vi "measureCombs_RF.vi"(3 "Read freqs. \nfrom textfile":bool=TRUE, 5 "Cluster":T2={"span"=600000000.0, "rbw"=1000.0, "enableVBW"=FALSE, "vbw"=0.0, "traceLength"=64001, "window"=0, "verticalUnit"=0, "center freq"=300000000.0} {"verticalUnit" items=["SpectrumVerticalUnit_dBm", "SpectrumVerticalUnit_Watt", "SpectrumVerticalUnit_Volt", "SpectrumVerticalUnit_Amp", "SpectrumVerticalUnit_dBmV"]; "window" items=["SpectrumWindow_Kaiser", "SpectrumWindow_Mil6dB", "SpectrumWindow_BlackmanHarris", "SpectrumWindow_Rectangle", "SpectrumWindow_FlatTop", "SpectrumWindow_Hann"]; "traceLength" items=["801"=801, "2401"=2401, "4001"=4001, "8001"=8001, "10401"=10401, "16001"=16001, "32001"=32001, "64001"=64001]}, 7 "RFC/ AFC measurement time":i32=30, 9 "Folder for all data (Don't forget the last slash!)":string) -> (0 "error out":errorcluster={"status"=TRUE, "code"=-1073807346, "source"="VISA Write in Agilent 33XXX Series.lvlib:Error Query.vi->Agilent 33XXX Series.lvlib:Close.vi->closeFncGen_AS.vi->measureCombs_anySet_keepAgilentOpen.vi"})   [LabVIEW 2016]
uses:
  <vilib>/Utility/file.llb/Read Delimited Spreadsheet (DBL).vi
  <vilib>/Utility/file.llb/Write Delimited Spreadsheet (DBL).vi
panel:
  in  "Agilent 33250A address":refnum<visa-resource-name>="GPIB0::4::INSTR"
  in  "Serial Configuration":T1={"Baud Rate"=9600, "Parity"=0, "Data Bits"=8, "Flow Control"=4} {"Flow Control" items=["None", "XON/XOFF", "RTS/CTS", "XON/XOFF & RTS/CTS", "DTR/DSR", "XON/XOFF & DTR/DSR"]; "Data Bits" items=["7"=7, "8"=8]; "Parity" items=["None", "Odd", "Even", "Mark", "Space"]; "Baud Rate" items=["300"=300, "600"=600, "1200"=1200, "2400"=2400, "4800"=4800, "9600"=9600, "19200"=19200]}
  in  "error in":errorcluster
  out "Last saved trace":sgl[](graph)
  in  "stop":bool
  out "RSA error out":errorcluster
  out "Real-time trace":sgl[](graph)
  out "Current set #":i32
  out "Current freq.":dbl=100000.0
  in  "freqs. file":path
  in  "Shuffle?":bool
  in  "Start freq":dbl=1000000.0 format="%0.2e"
  in  "End freq":dbl=2000000.0 format="%0.2e"
  in  "Freq step":i32=100000 format="%.2e"
  out "Duration array":T3(array[cluster])
  in  "Mod shape":enum16{"Triangle", "Sine"}(ring)
  # "consecutive sweeps can be compared\nto check for probe on AFC."
  # "RSA settings"
  # "Suppose you want to collect comb data, first ascending, then descending.\n\nIn Matlab, create a 1xM array \ncontaining all modulation freqs (Hz) in the ascending sequence; then create a 1xN array for the descending case. Note that M != N is fine.\n\nfid= fopen(FILENAME, 'w');\nfprintf(fid,'%d\\t', ARRAY1);\nfprintf(fid,'\\r\\n');\nfprintf(fid,'%d\\t',ARRAY2);\n... \n(for more sets, repeat as needed)\nfclose(fid);\n\nNow find the file you just made:"
  # "Modulation settings"
  # "(zero-indexed)"
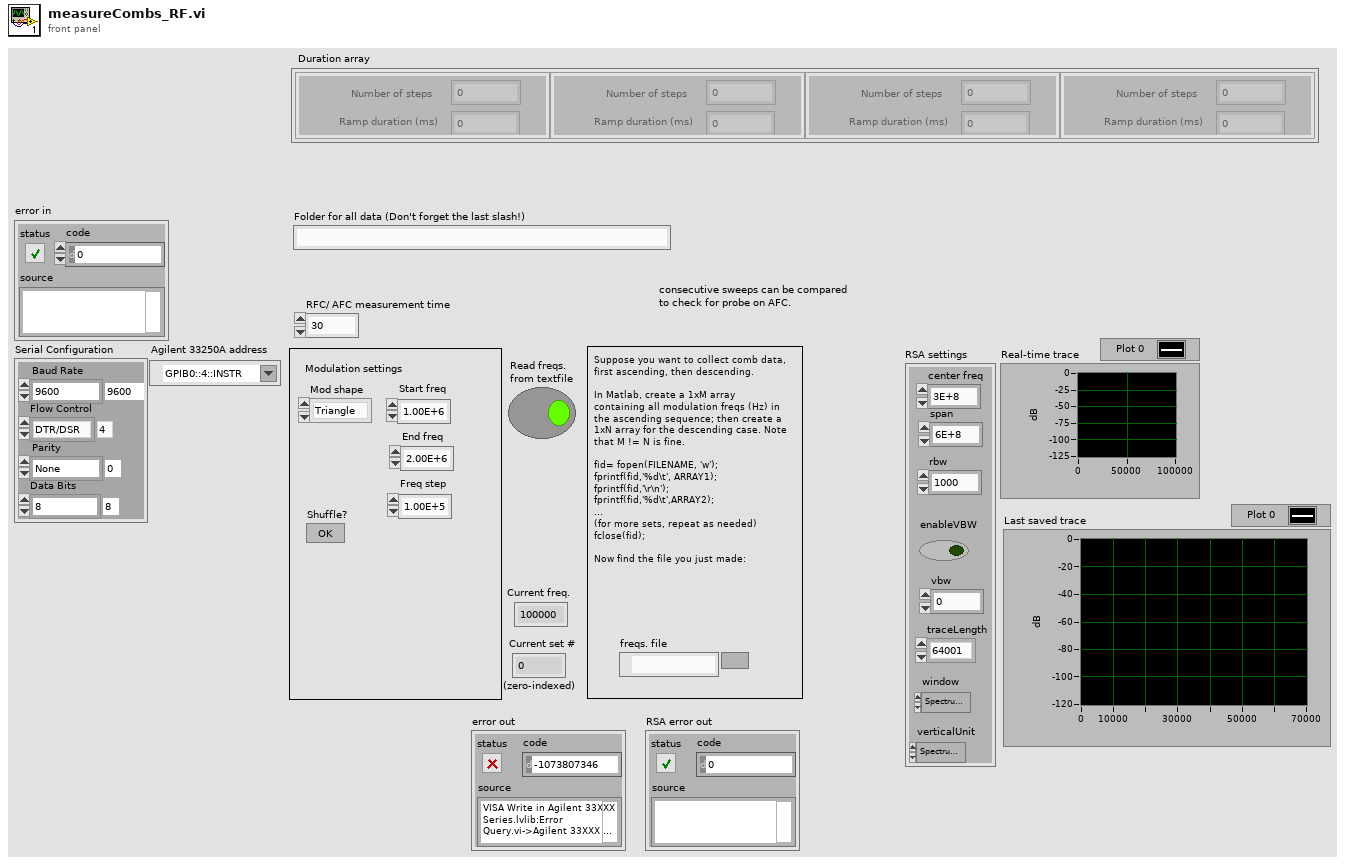
[diagram p1: front panel]
types:
  T1 = cluster{"Baud Rate":u32, "Parity":u16, "Data Bits":u16, "Flow Control":u16}
  T2 = cluster{"span":dbl, "rbw":dbl, "enableVBW":bool, "vbw":dbl, "traceLength":u16, "window":u32, "verticalUnit":u32, "center freq":dbl}
  T3 = cluster{"Number of steps":dbl, "Ramp duration (ms)":dbl}[]
  T4 = cluster{"span":dbl, "rbw":dbl, "enableVBW":bool, "vbw":dbl, "traceLength":u16, "window":u32, "verticalUnit":u32}
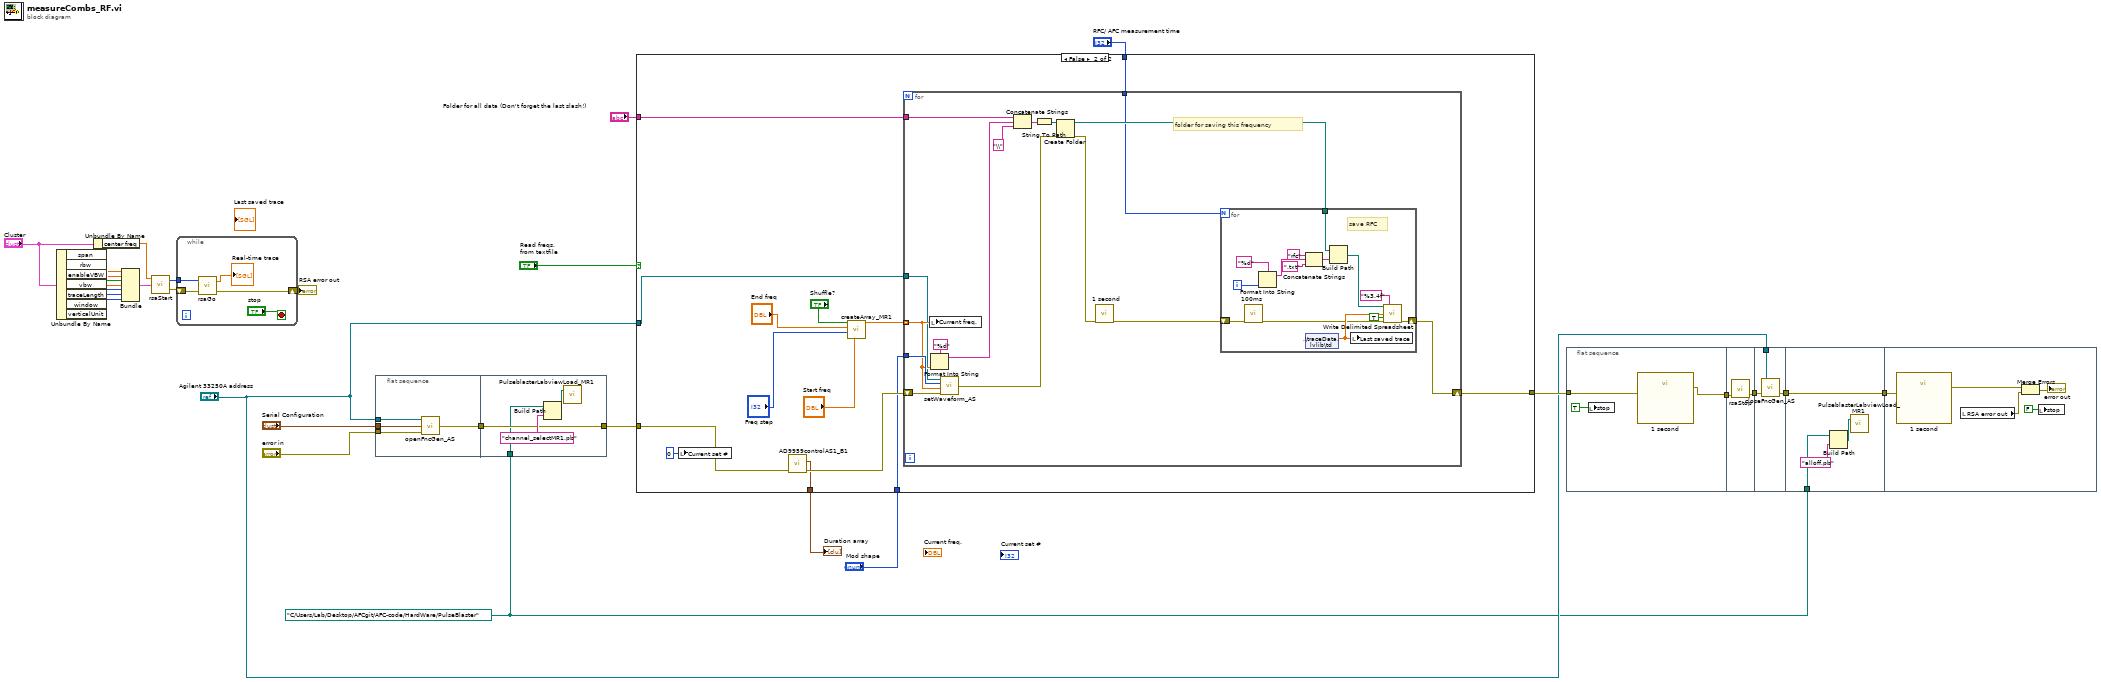
[diagram p0: block diagram]
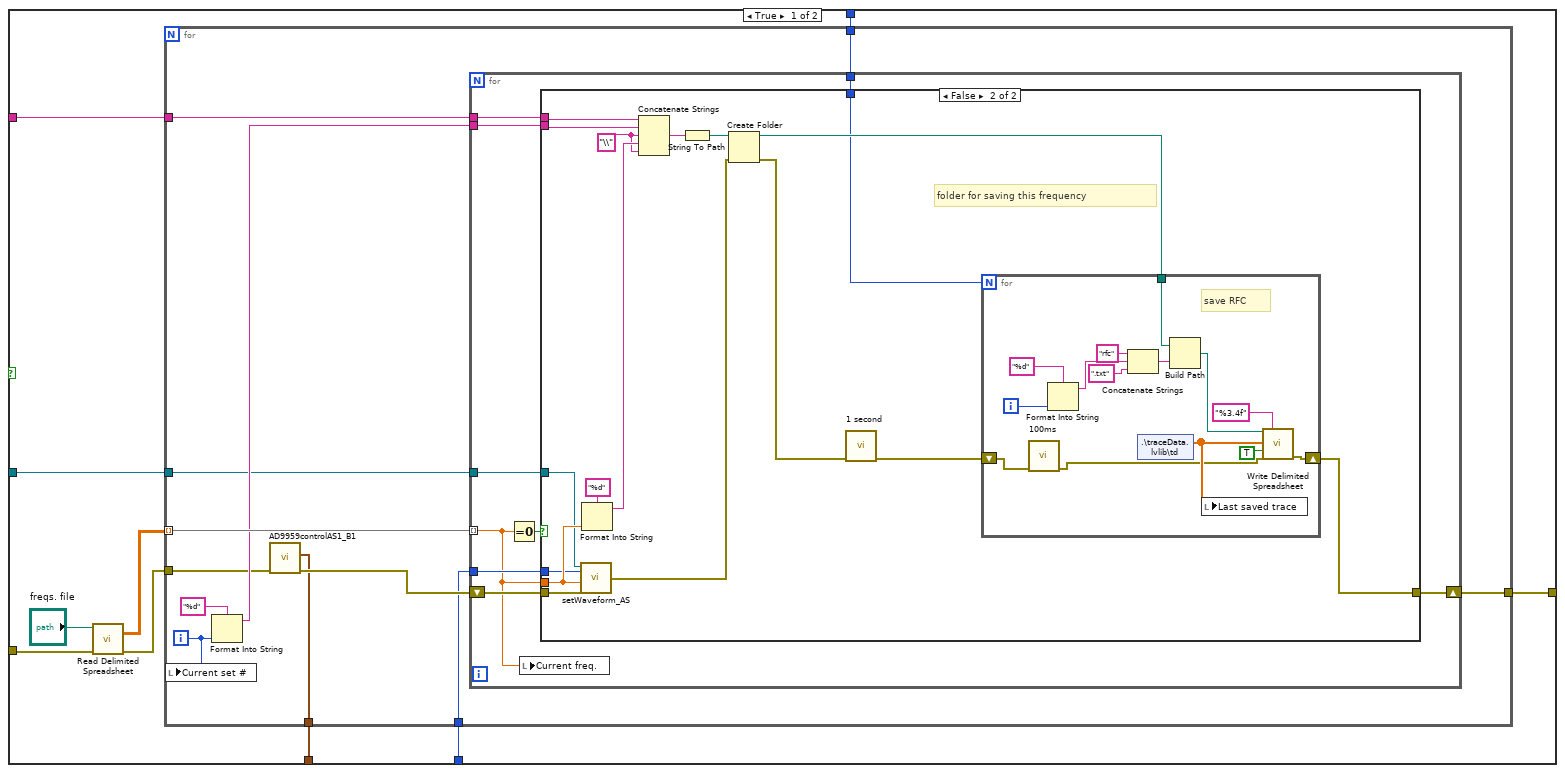
[diagram p2: hidden frame]
diagram:
  w1 = path "C:/Users/Lab/Desktop/AFCgit/AFC-code/HardWare/PulseBlaster" ("base path")
  n1 = Unbundle By Name("Cluster") -> ("span"=w22:dbl, "rbw"=w23:dbl, "enableVBW"=w24:bool, "vbw"=w25:dbl, "traceLength"=w26:u16, "window"=w27:u32, "verticalUnit"=w28:u32)
  n2 = Unbundle By Name("Cluster") -> ("center freq"=w16:dbl)
  n3 = Bundle("span"=w22, "rbw"=w23, "enableVBW"=w24, "vbw"=w25, "traceLength"=w26, "window"=w27, "verticalUnit"=w28) -> (w15:T4)  [unwired: 1 in]
  n4 = call "rsaStart.vi"("Cluster"=w15, "center freq"=w16) -> ("error out"=w13:errorcluster, "traceLength"=w14:u16)  [unwired: 1 in]
  n5 = while {
    tunnel: w14 -> [w34]
    shift-right: [w32] -> w12
    shift-left: w13 -> [w31]
    stop <- "stop" stop-if-true
    n6 = call "rsaGo.vi"("error in"=w31, "Trace length"=w34) -> ("error out"=w32:errorcluster, "traceData out"=→"Real-time trace":sgl[])  [unwired: 1 in]
  }
  "RSA error out" <- w12
  n7 = flat-sequence {
    tunnel: "error in" -> [w38]
    tunnel: "Serial Configuration" -> [w37]
    tunnel: "Agilent 33250A address" -> [w36]
    tunnel: [w35] -> w3
    tunnel: [w40] -> w2
    tunnel: w3 -> [w40]
    tunnel: w1 -> [w39]
    frame #0 {
      n8 = call "openFncGen_AS.vi"("error in (no error)"=w38, "Serial Configuration"=w37, "VISA resource name"=w36) -> ("error out"=w35:errorcluster)
    }
    frame #1 {
      n9 = Build Path(base path=w39, name or relative path="channel_selectMR1.pb") -> (appended path=w42:path)
      n10 = call "PulseblasterLabviewLoad_MR1.vi"("Input file"=w42) -> ()  [unwired: 1 in, 2 out]
    }
  }
  n11 = case shown="False" "Read freqs. \nfrom textfile" {
    tunnel: "Folder for all data (Don't forget the last slash!)" -> [w52 w119]
    tunnel: "RFC/ AFC measurement time" -> [w51 w117]
    tunnel: w2 -> [w49 w111]
    tunnel: "Mod shape" -> [w46 w110]
    tunnel: [w45 w109] -> w17
    tunnel: [w44 w107] -> w29
    tunnel: "Agilent 33250A address" -> [w43 w106]
    frame True {
      n12 = call-poly <vilib>:"Read Delimited Spreadsheet.vi"("file path (dialog if empty)"="freqs. file", "error in (no error)"=w49) -> ("all rows"=w48:dbl[][], "error out"=w47:errorcluster)  [unwired: 8 in, 4 out]
      n13 = for {
        tunnel: [w64] -> w44
        tunnel: w52 -> [w63]
        tunnel: w51 -> [w61]
        tunnel: w48 -> [w60] mode=indexing
        tunnel: w47 -> [w57]
        tunnel: w46 -> [w56]
        tunnel: [w55] -> w45
        tunnel: w43 -> [w53]
        i -> [w54]
        n14 = local write "Current set #"(w54) -> ()
        n15 = Format Into String(format string="%d", w54) -> (resulting string=w58:string)  [unwired: 2 in, 1 out]
        n16 = call "AD9959controlAS1_B1.vi"("error in (no error)"=w57) -> ("error out"=w62:errorcluster, "Duration array"=w55:T3)  [unwired: 9 in]
        n17 = for {
          tunnel: w60 -> [w66] mode=indexing
          tunnel: w56 -> [w73]
          shift-right: [w72] -> w64
          shift-left: w62 -> [w71]
          tunnel: w63 -> [w68]
          tunnel: w61 -> [w70]
          tunnel: w58 -> [w69]
          tunnel: w53 -> [w65]
          n18 = Equal To 0?(x=w66) -> (x = 0?=w67:bool)
          n19 = local write "Current freq."(w66) -> ()
          n20 = case shown="False" w67 {
            tunnel: w73 -> [_ w79]
            tunnel: [w74 w75] -> w72
            tunnel: w71 -> [w74 w81]
            tunnel: w70 -> [_ w89]
            tunnel: w69 -> [_ w84]
            tunnel: w68 -> [_ w85]
            tunnel: w66 -> [_ w80]
            tunnel: w65 -> [_ w78]
            frame True {
            }
            frame False {
              w87 = "\\" ("string")
              # "folder for saving this frequency"
              n21 = call "setWaveform_AS.vi"("error in (no error)"=w81, "Frequency (1000 Hz)"=w80, "Enum"=w79, "VISA resource name"=w78) -> ("error out"=w76:errorcluster)
              n22 = Format Into String(format string="%d", w80) -> (resulting string=w88:string)  [unwired: 2 in, 1 out]
              n23 = Concatenate Strings(w85, w84, w87, w88, w87) -> (w83:string)
              n24 = String To Path(string=w83) -> (path=w90:path)
              n25 = Create Folder(path (use dialog)=w90, error in=w76) -> (created path=w91:path, error out=w77:errorcluster)  [unwired: 1 in, 1 out]
              n26 = call "1 second"("error in (no error)"=w77) -> ("error out"=w82:errorcluster)  [unwired: 10 in]
              n27 = for {
                N: w89 -> [_]
                shift-right: [w104] -> w75
                shift-left: w82 -> [w93]
                tunnel: w91 -> [w96]
                i -> [w100]
                # "save RFC"
                n28 = call "100ms"("error in (no error)"=w93) -> ("error out"=w92:errorcluster)  [unwired: 10 in]
                n29 = Format Into String(format string="%d", w100) -> (resulting string=w99:string)  [unwired: 2 in, 1 out]
                n30 = Concatenate Strings("rfc" ("string"), w99, ".txt" ("string")) -> (w98:string)
                n31 = shared-variable ".\\traceData.lvlib\\td"() -> (w94:dbl[])  [unwired: 1 in, 1 out]
                n32 = Build Path(base path=w96, name or relative path=w98) -> (appended path=w103:path)
                n33 = local write "Last saved trace"(w94) -> ()
                n34 = call-poly <vilib>:"Write Delimited Spreadsheet.vi"("file path (dialog if empty)"=w103, "format (%.3f)"="%3.4f", "1D data"=w94, "append to file? (new file:F)"=TRUE, "error in (no error)"=w92) -> ("error out"=w104:errorcluster)  [unwired: 9 in, 1 out]
              }
            }
          }
        }
      }
    }
    frame False {
      n35 = local write "Current set #"(0 ("Current set #")) -> ()
      n36 = call "AD9959controlAS1_B1.vi"("error in (no error)"=w111) -> ("error out"=w118:errorcluster, "Duration array"=w109:T3)  [unwired: 9 in]
      n37 = call "createArray_MR1.vi"("Start freq"="Start freq", "Freq step"="Freq step", "End freq"="End freq", "Shuffle?"="Shuffle?") -> ("Riffled {X}"=w112:dbl[])  [unwired: 7 in]
      n38 = for {
        tunnel: w112 -> [w125] mode=indexing
        tunnel: w110 -> [w126]
        shift-right: [w120] -> w107
        shift-left: w118 -> [w127]
        tunnel: w119 -> [w130]
        tunnel: w117 -> [w129]
        tunnel: w106 -> [w124]
        # "folder for saving this frequency"
        n39 = local write "Current freq."(w125) -> ()
        n40 = Format Into String(format string="%d", w125) -> (resulting string=w134:string)  [unwired: 2 in, 1 out]
        n41 = call "setWaveform_AS.vi"("error in (no error)"=w127, "Frequency (1000 Hz)"=w125, "Enum"=w126, "VISA resource name"=w124) -> ("error out"=w121:errorcluster)
        n42 = Concatenate Strings(w130, w134, "\\" ("string")) -> (w132:string)
        n43 = String To Path(string=w132) -> (path=w131:path)
        n44 = Create Folder(path (use dialog)=w131, error in=w121) -> (created path=w133:path, error out=w123:errorcluster)  [unwired: 1 in, 1 out]
        n45 = call "1 second"("error in (no error)"=w123) -> ("error out"=w122:errorcluster)  [unwired: 10 in]
        n46 = for {
          N: w129 -> [_]
          shift-right: [w148] -> w120
          shift-left: w122 -> [w137]
          tunnel: w133 -> [w140]
          i -> [w144]
          # "save RFC"
          n47 = call "100ms"("error in (no error)"=w137) -> ("error out"=w136:errorcluster)  [unwired: 10 in]
          n48 = Format Into String(format string="%d", w144) -> (resulting string=w143:string)  [unwired: 2 in, 1 out]
          n49 = Concatenate Strings("rfc" ("string"), w143, ".txt" ("string")) -> (w142:string)
          n50 = shared-variable ".\\traceData.lvlib\\td"() -> (w138:dbl[])  [unwired: 1 in, 1 out]
          n51 = Build Path(base path=w140, name or relative path=w142) -> (appended path=w147:path)
          n52 = local write "Last saved trace"(w138) -> ()
          n53 = call-poly <vilib>:"Write Delimited Spreadsheet.vi"("file path (dialog if empty)"=w147, "format (%.3f)"="%3.4f", "1D data"=w138, "append to file? (new file:F)"=TRUE, "error in (no error)"=w136) -> ("error out"=w148:errorcluster)  [unwired: 9 in, 1 out]
        }
      }
    }
  }
  "Duration array" <- w17
  n54 = flat-sequence {
    tunnel: w29 -> [w151]
    tunnel: [w150] -> w11
    tunnel: w11 -> [w154]
    tunnel: [w153] -> w9
    tunnel: w9 -> [w156]
    tunnel: [w157] -> w8
    tunnel: "Agilent 33250A address" -> [w155]
    tunnel: w8 -> [w159]
    tunnel: [w159] -> w7
    tunnel: w1 -> [w158]
    tunnel: w7 -> [w163]
    frame #0 {
      n55 = local write "stop"(TRUE ("Stop")) -> ()
      n56 = call "1 second"("error in (no error)"=w151) -> ("error out"=w150:errorcluster)  [unwired: 10 in]
    }
    frame #1 {
      n57 = call "rsaStop.vi"("error in (no error)"=w154) -> ("error out"=w153:errorcluster)  [unwired: 3 in]
    }
    frame #2 {
      n58 = call "closeFncGen_AS.vi"("error in (no error)"=w156, "VISA resource name"=w155) -> ("error out"=w157:errorcluster)  [unwired: 1 in]
    }
    frame #3 {
      n59 = Build Path(base path=w158, name or relative path="alloff.pb") -> (appended path=w161:path)
      n60 = call "PulseblasterLabviewLoad_MR1.vi"("Input file"=w161) -> ()  [unwired: 1 in, 2 out]
    }
    frame #4 {
      n61 = call "1 second"("error in (no error)"=w163) -> ("error out"=w162:errorcluster)  [unwired: 10 in]
      n62 = local read "RSA error out"() -> (w166:errorcluster)
      n63 = Merge Errors(w162, w166) -> (→"error out":errorcluster)
      n64 = local write "stop"(FALSE ("stop")) -> ()
    }
  }
